vi "AAA Test Case, Catalog.vi"   [LabVIEW 2010]
panel:
  # "Test Case\nCatalog"
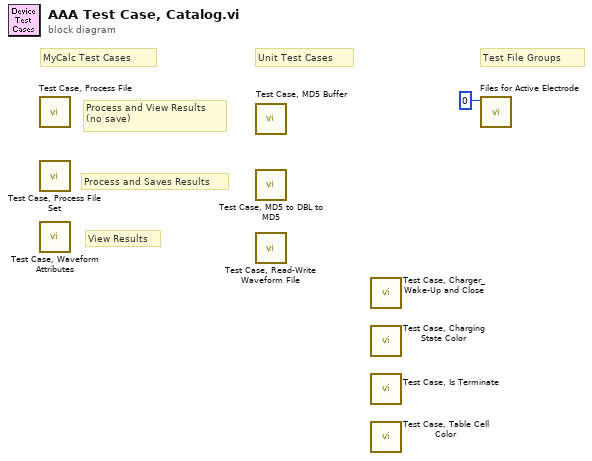
[diagram p0: block diagram]
diagram:
  # "Process and View Results\n(no save)"
  # "View Results"
  # "Process and Saves Results"
  # "Unit Test Cases"
  # "Test File Groups"
  # "MyCalc Test Cases"
  n1 = call "Test Case, Process File.vi"() -> ()  [unwired: 8 in, 4 out]
  n2 = call "Test Case, Process File Set.vi"() -> ()  [unwired: 8 in, 4 out]
  n3 = call "Test Case, Waveform Attributes.vi"() -> ()  [unwired: 12 in]
  n4 = call "Test Case, MD5 Buffer.vi"() -> ()  [unwired: 12 in]
  n5 = call "Test Case, MD5 to DBL to MD5.vi"() -> ()  [unwired: 12 in]
  n6 = call "Test Case, Read-Write Waveform File.vi"() -> ()  [unwired: 12 in]
  n7 = call "Test Case, Charger_Wake-Up and Close.vi"() -> ()  [unwired: 7 in, 1 out]
  n8 = call "Test Case, Charging State Color.vi"() -> ()  [unwired: 12 in]
  n9 = call "Test Case, Is Terminate.vi"() -> ()  [unwired: 12 in]
  n10 = call "Test Case, Table Cell Color.vi"() -> ()  [unwired: 12 in]
  n11 = call "Files for Active Electrode.vi"("index"=0) -> ()  [unwired: 4 in, 5 out]
